vi "Image.vi"(2 "XRef":refnum<vi>, 3 "State In":T1) -> (0 "Image":picture)   [LabVIEW 2010, in "CData Flatten XNode.xnode"]
doc: "This ability VI is used to describe your XNode's appearance. The origin of Image corresponds to the top-left corner of your XNode. The bounds of your XNode are used to crop this image. If you want LabVIEW to update your image, you need to inform it through the UpdateImage or UpdateImageAndBounds replies. Any areas where you do not draw are transparent, so regions intended to appear white should be explicitly drawn.\n \n Remember to localize any strings that are part of your image.\n\nDefault behavior: None.\n\nThis ability does not provide UI and OS messages are not handled."
uses:
  CData Flatten XNode.xnode
  State.ctl
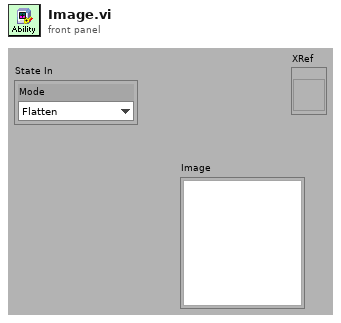
[diagram p1: front panel]
types:
  T1 = typedef "CData Flatten XNode.xnode/State.ctl" = cluster{"Mode":enum16{"Flatten", "Unflatten"}}
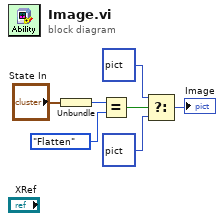
[diagram p0: block diagram]
diagram:
  n1 = Unbundle("State In") -> ("Mode"=w6:enum16{"Flatten", "Unflatten"})
  n2 = Equal?(x=w6, y=enum16{"Flatten", "Unflatten"}."Flatten") -> (x = y?=w4:bool)
  n3 = Select(t=picture bytes[3230] ("new picture"), s=w4, f=picture bytes[3230] ("new picture")) -> (s? t:f=→"Image":picture)
